vi "Unflatten-SensorEventData.vi"(8 "error in (no error)":errorcluster, 11 "Event Binary Data":string) -> (0 "error out":errorcluster, 3 "Event Data":T1)   [LabVIEW 2026, in "SDL3.lvlib" / "Events.lvlib"]
uses:
  SensorEventData--cluster.ctl
  Joystick/JoystickID--integer.ctl
  Sensor/SensorID--integer.ctl
  Events.lvlib
  Joystick/Joystick.lvlib
  Sensor/Sensor.lvlib
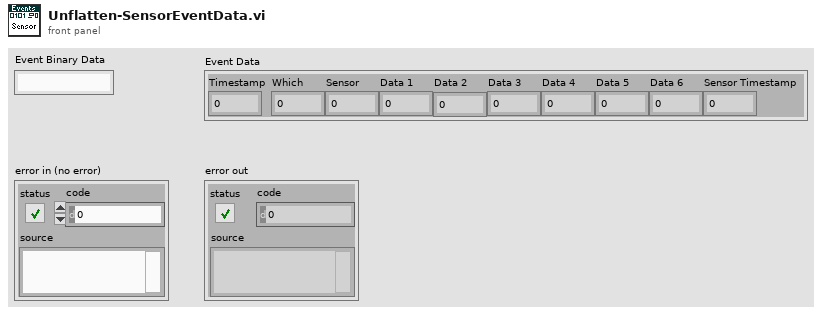
[diagram p1: front panel]
types:
  T1 = typedef "SDL3.lvlib/Events.lvlib/SensorEventData--cluster.ctl" = cluster{"Timestamp":u64, "Which":T2, "Sensor":T3, "Data 1":sgl, "Data 2":sgl, "Data 3":sgl, "Data 4":sgl, "Data 5":sgl, "Data 6":sgl, "Sensor Timestamp":u64}
  T2 = typedef "SDL3.lvlib/Joystick.lvlib/JoystickID--integer.ctl" = u32
  T3 = typedef "SDL3.lvlib/Sensor.lvlib/SensorID--integer.ctl" = u32
  T4 = enum16{"big-endian, network order", "native, host order", "little-endian"}
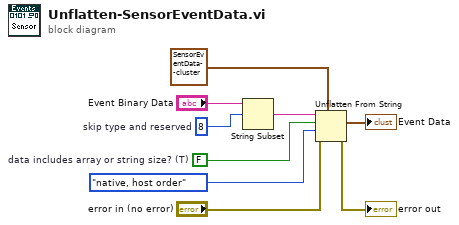
[diagram p0: block diagram]
diagram:
  w3 = 8  # skip type and reserved
  w6 = FALSE  # data includes array or string size? (T)
  n1 = String Subset(string="Event Binary Data", offset (0)=w3) -> (substring=w4:string)  [unwired: 1 in]
  n2 = Unflatten From String(type=T1 {"Timestamp"=0, "Which"=0, "Sensor"=0, "Data 1"=0.0, "Data 2"=0.0, "Data 3"=0.0, "Data 4"=0.0, "Data 5"=0.0, "Data 6"=0.0, "Sensor Timestamp"=0} ("SensorEvent"), binary string=w4, data includes array or string size? (T)=w6, byte order (0:big-endian, network order)=T4."native, host order", error in (no error)="error in (no error)") -> (value=→"Event Data":T1, error out=→"error out":errorcluster)  [unwired: 1 out]
